vi "Read Warming.vi"(8 "error in (no error)":errorcluster, 11 "In":refnum<class "Sim Laser Driver.lvclass">) -> (0 "error out":errorcluster, 2 "Warming":bool, 3 "Out":refnum<class "Sim Laser Driver.lvclass">)   [LabVIEW 2022 SP3, in "Sim Laser Driver.lvclass"]
uses:
  Sim Laser Driver.lvclass
  Sim Laser Driver.lvclass/Sim Laser Driver.ctl
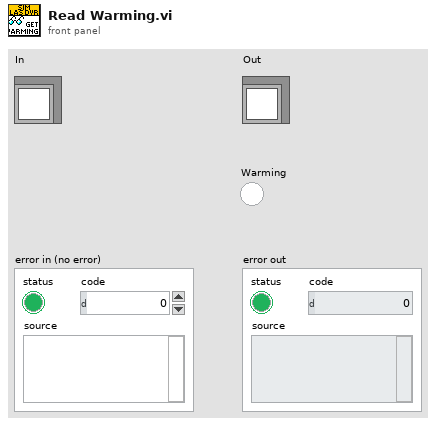
[diagram p1: front panel]
types:
  T1 = typedef "Sim Laser Driver.lvclass/data.ctl" = cluster{"Settings":T2, "Warming":bool, "Firing":bool, "Current Temp":dbl}
  T2 = typedef "Sim Laser Driver.lvclass/settings.ctl" = cluster{"Power":dbl}
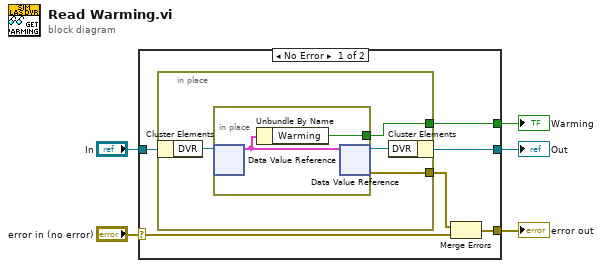
[diagram p0: block diagram]
diagram:
  n1 = case shown="No Error" "error in (no error)" {
    selector: "error in (no error)" -> [w6 w19]
    tunnel: [w7 w19] -> w4
    tunnel: [w11 w18] -> w3
    tunnel: "In" -> [w10 w18]
    tunnel: [w9 _] -> w1
    frame No Error {
      n2 = in-place {
        in-place-border: [w13] -> w9
        in-place-border: [w12] -> w8
        n3 = in-place-cluster #1(w10) -> ("DVR"=w14:refnum<data-value>)
        n4 = in-place {
          in-place-border: [w16] -> w13
          n5 = in-place-dvr #2(w14) -> (w17:T1)  [unwired: 1 out]
          n6 = Unbundle By Name(w17) -> ("Warming"=w16:bool)
          n7 = in-place-dvr #2(w17) -> (w15:refnum<data-value>, w12:errorcluster)
        }
        n8 = in-place-cluster #1("DVR"=w15) -> (w11:refnum<class "Sim Laser Driver.lvclass">)
      }
      n9 = Merge Errors(w8, w6) -> (w7:errorcluster)
    }
    frame Error {
    }
  }
  "Out" <- w3
  "error out" <- w4
  "Warming" <- w1
